vi "Test Empty Invalid Null.vi"() -> ()   [LabVIEW 2017]
uses:
  JSONtext.lvlib
  <vilib>/addons/_JKI Toolkits/Caraya/classes/Test/Test.lvclass
  <vilib>/addons/_JKI Toolkits/Caraya/classes/Assert/Assert.lvclass
panel:
  out "Not Null/empty Invalid":bool[](array[boolean])
  out "Null, Empty or Invalid":bool[](array[boolean])
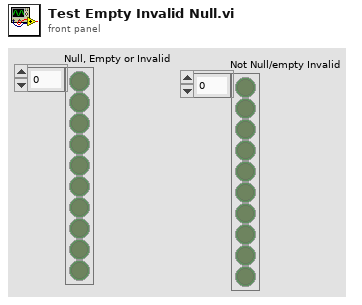
[diagram p1: front panel]
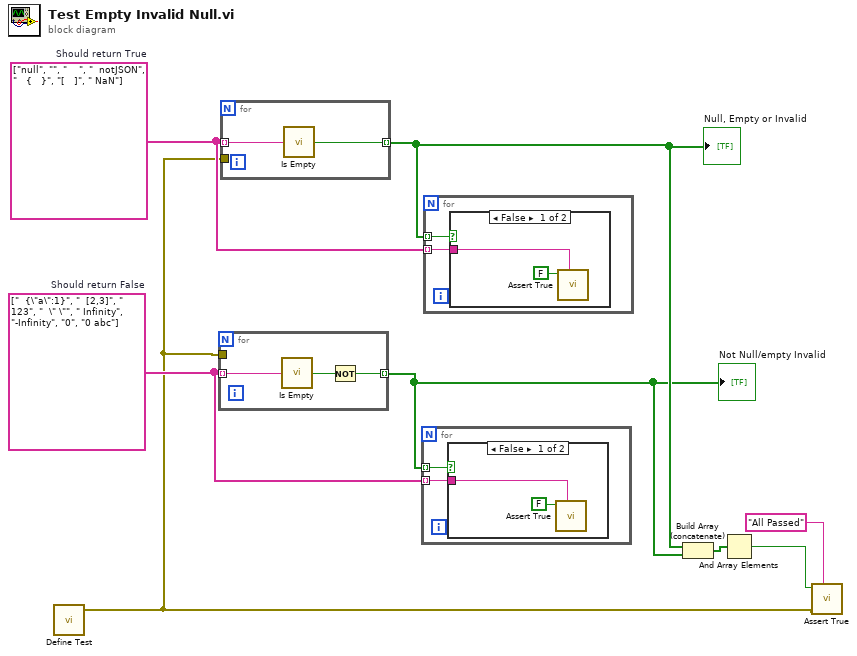
[diagram p0: block diagram]
diagram:
  w4 = string[] ["  {\"a\":1}", "  [2,3]", "    123", "  \" \"", " Infinity", "-Infinity", "0", "0 abc"]  # Should return False
  w5 = string[] ["null", "", "    ", "  notJSON", "   {   }", "[   ]", " NaN"]  # Should return True
  n1 = call <vilib>:"Define Test.vi"() -> ("error out"=w1:errorcluster)  [unwired: 11 in]
  n2 = for {
    tunnel: w4 -> [w11] mode=indexing
    tunnel: [w9] -> w2 mode=indexing
    tunnel: w1 -> [_]
    n3 = call "Is Empty.vi"("JSON"=w11) -> ("Null, Empty or Invalid"=w10:bool)  [unwired: 4 in]
    n4 = Not(x=w10) -> (.not. x?=w9:bool)
  }
  "Not Null/empty Invalid" <- w2
  n5 = for {
    tunnel: w5 -> [w13] mode=indexing
    tunnel: [w12] -> w6 mode=indexing
    tunnel: w1 -> [_]
    n6 = call "Is Empty.vi"("JSON"=w13) -> ("Null, Empty or Invalid"=w12:bool)  [unwired: 4 in]
  }
  "Null, Empty or Invalid" <- w6
  n7 = for {
    tunnel: w2 -> [w15] mode=indexing
    tunnel: w4 -> [w14] mode=indexing
    n8 = case shown="False" w15 {
      tunnel: w14 -> [w17 _]
      frame False {
        n9 = call <vilib>:"Assert True.vi"("Label"=w17, "True?"=FALSE) -> ()  [unwired: 9 in, 1 out]
      }
      frame True {
      }
    }
  }
  n10 = for {
    tunnel: w6 -> [w19] mode=indexing
    tunnel: w5 -> [w18] mode=indexing
    n11 = case shown="False" w19 {
      tunnel: w18 -> [w21 _]
      frame False {
        n12 = call <vilib>:"Assert True.vi"("Label"=w21, "True?"=FALSE) -> ()  [unwired: 9 in, 1 out]
      }
      frame True {
      }
    }
  }
  n13 = Build Array (concatenate)(w6, w2) -> (w3:bool[])
  n14 = And Array Elements(Boolean array=w3) -> (logical AND=w7:bool)
  n15 = call <vilib>:"Assert True.vi"("Label"="All Passed", "error in (no error)"=w1, "True?"=w7) -> ()  [unwired: 8 in, 1 out]
